vi "V&V Basic Transmit.vi"() -> ()   [LabVIEW 2012, in "UART_Host_Driver.lvlib" / "UART Driver.lvclass"]
doc: "This example calls the UART Initialize, UART Configure Port, UART Execute Command, and a UART Close."
uses:
  UART Driver.lvclass
  Typedefs/Configuration Parameters.ctl
  FPGA/UART/StopBits.ctl
  FPGA/UART/Parity.ctl
  <vilib>/Instr/_visa.llb/VISA Configure Serial Port (Instr).vi
  FPGA/UART/UART_Firmware.lvlib
  UART_Host_Driver.lvlib
panel:
  out "Rx Data":string
  out "Number of Reads Executed":i32
  out "Number of Read Errors":i32
  in  "stop":bool
  in  "Configuration Parameters":T1={"Baud"=115200, "Character Length"=8, "Stop Bits"=enum."1.0", "Parity"=enum."None", "Character Spacing (ticks)"=0}
  in  "Tx Data":string="TEST"
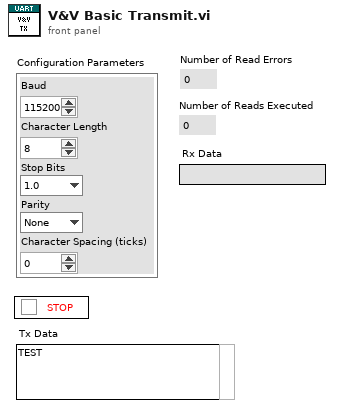
[diagram p1: front panel]
types:
  T1 = typedef "UART_Host_Driver.lvlib/Configuration Parameters.ctl" = cluster{"Baud":u32, "Character Length":u8, "Stop Bits":T2, "Parity":T3, "Character Spacing (ticks)":u32}
  T2 = typedef "UART_Firmware.lvlib/StopBits.ctl" = enum8{"1.0", "1.5", "2.0"}
  T3 = typedef "UART_Firmware.lvlib/Parity.ctl" = enum8{"None", "Even", "Odd"}
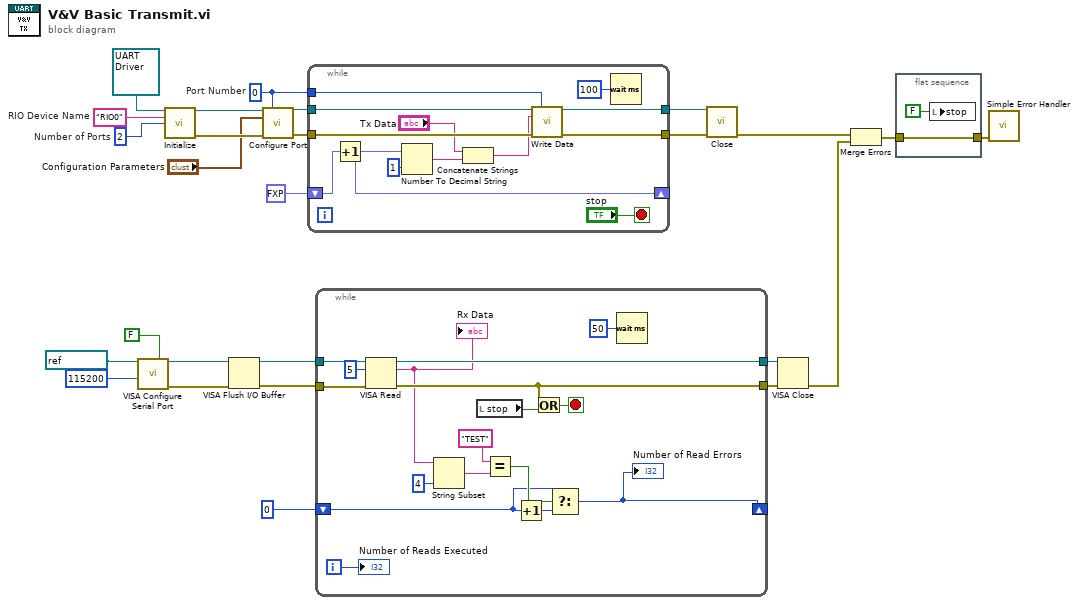
[diagram p0: block diagram]
diagram:
  w18 = u8 0  # Port Number
  w22 = u8 2  # Number of Ports
  w23 = "RIO0"  # RIO Device Name
  n1 = call-poly "VISA Configure Serial Port"("VISA resource name"=refnum<visa-resource-name> "COM1", "Enable Termination\nChar (T)"=FALSE ("Enable Termination\nChar (T)"), "baud rate (9600)"=u32 115200) -> ("VISA resource name out"=w7:refnum<visa-resource-name>, "error out"=w6:errorcluster)  [unwired: 11 in]
  n2 = call-dynamic "Initialize.vi"("UART Driver in"=refnum<class "UART Driver.lvclass"> refnum, "RIO Device Name"=w23, "Number of UART Controllers"=w22) -> ("UART Driver out"=w26:refnum<class "UART Driver.lvclass">, "error out"=w25:errorcluster)  [unwired: 11 in]
  n3 = VISA Flush I/O Buffer(VISA resource name=w7, error in (no error)=w6) -> (VISA resource name out=w4:refnum<visa-resource-name>, error out=w5:errorcluster)  [unwired: 1 in]
  n4 = call-dynamic "Configure Port.vi"("UART Driver in"=w26, "Controller Number"=w18, "Configuration Parameters"="Configuration Parameters", "error in"=w25) -> ("UART Driver out"=w20:refnum<class "UART Driver.lvclass">, "error out"=w19:errorcluster)  [unwired: 10 in]
  n5 = while {
    tunnel: w20 -> [w39]
    tunnel: w19 -> [w38]
    tunnel: w18 -> [w37]
    tunnel: [w36] -> w17
    tunnel: [w35] -> w16
    shift-right: [w27] -> _
    shift-left: fxp<+,3,3> 0.0 -> [w29]
    stop <- "stop" stop-if-true
    n6 = Increment(x=w29) -> (x+1=w27:fxp<+,3,3>)
    n7 = Number To Decimal String(number=w27, width (-)=i16 1) -> (decimal integer string=w30:string)
    n8 = Concatenate Strings("Tx Data", w30) -> (w31:string)
    n9 = call-dynamic "Write Data.vi"("UART Driver in"=w39, "Port Number"=w37, "Tx Data"=w31, "error in"=w38) -> ("UART Driver out"=w35:refnum<class "UART Driver.lvclass">, "error out"=w36:errorcluster)  [unwired: 10 in]
    n10 = Wait (ms)(milliseconds to wait=u32 100) -> ()  [unwired: 1 out]
  }
  n11 = while {
    tunnel: w5 -> [w55]
    tunnel: w4 -> [w56]
    tunnel: [w51] -> w11
    tunnel: [w50] -> w12
    shift-right: [w42] -> _
    shift-left: 0 -> [w44]
    i -> [w41]
    stop <- w53 stop-if-true
    n12 = VISA Read(VISA resource name=w56, byte count=u32 5, error in (no error)=w55) -> (VISA resource name out=w50:refnum<visa-resource-name>, read buffer=w40:string, error out=w51:errorcluster)  [unwired: 1 out]
    "Rx Data" <- w40
    n13 = String Subset(string=w40, length (rest)=4 ("length (rest)")) -> (substring=w47:string)  [unwired: 1 in]
    n14 = local read "stop"() -> (w52:bool)
    n15 = Equal?(x="TEST", y=w47) -> (x = y?=w45:bool)
    n16 = Increment(x=w44) -> (x+1=w43:i32)
    n17 = Or(x=w51, y=w52) -> (x .or. y?=w53:bool)
    n18 = Select(t=w44, s=w45, f=w43) -> (s? t:f=w42:i32)
    "Number of Read Errors" <- w42
    n19 = Wait (ms)(milliseconds to wait=u32 50) -> ()  [unwired: 1 out]
    "Number of Reads Executed" <- w41
  }
  n20 = call-dynamic "Close.vi"("UART Driver in"=w16, "error in"=w17) -> ("error out"=w10:errorcluster)  [unwired: 13 in]
  n21 = VISA Close(VISA resource name=w12, error in (no error)=w11) -> (error out=w9:errorcluster)
  n22 = Merge Errors(w10, w9) -> (w3:errorcluster)
  n23 = flat-sequence {
    tunnel: w3 -> [w58]
    tunnel: [w58] -> w2
    frame #0 {
      n24 = local write "stop"(FALSE ("stop")) -> ()
    }
  }
  n25 = call <vilib>:"Simple Error Handler.vi"("error in (no error)"=w2) -> ()  [unwired: 4 in, 5 out]
